vi "RSZVB Set TDIF Amplitude Imbalance Stop Power.vi"(8 "error in (no error)":errorcluster {"code" format="%.0x"}, 9 "Stop Power (+10.0 dBm)":dbl=10.0 format="%^.3e", 10 "Channel (1)":i32=1, 11 "VISA session":refnum<visa-resource-name>) -> (0 "error out":errorcluster {"code" format="%.0x"}, 3 "dup VISA session":refnum<visa-resource-name>)   [LabVIEW 2011]
doc: "This VI defines the stop power for an amplitude imbalance sweep, which is equal to the right edge of a Cartesian diagram. A balanced port configuration must be defined and an amplitude imbalance sweep must be active to use this VI.\n\nNote(s):\n\n(1) This VI is available only with option R&S ZVA-K6.\n\nRemote-control command(s):\nSOURce<Ch>:TDIF:IMBalance:AMPLitude:STOP <stop_power>"
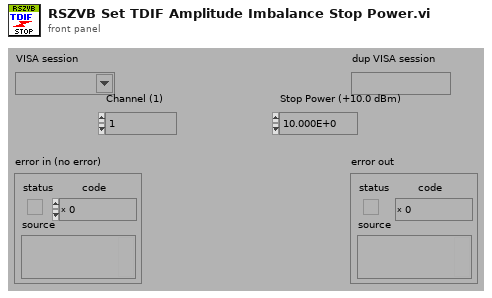
[diagram p1: front panel]
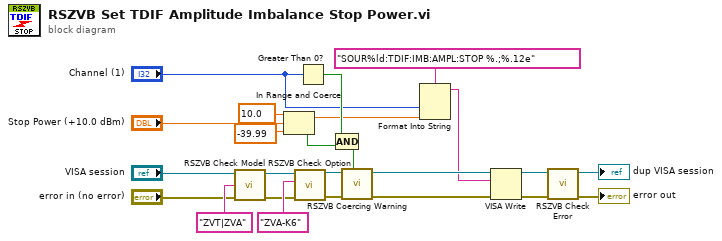
[diagram p0: block diagram]
diagram:
  n1 = call "RSZVB Check Model.vi"("error in (no error)"="error in (no error)", "Model"="ZVT|ZVA" ("Options"), "VISA session"="VISA session") -> ("error out"=w21:errorcluster, "dup VISA session"=w22:refnum<visa-resource-name>)  [unwired: 7 in]
  n2 = In Range and Coerce(upper limit=10.0, x="Stop Power (+10.0 dBm)", lower limit=-39.99) -> (coerced(x)=w9:dbl, In Range?=w16:bool)
  n3 = call "RSZVB Check Option.vi"("error in (no error)"=w21, "Options"="ZVA-K6", "VISA session"=w22) -> ("error out"=w8:errorcluster, "dup VISA session"=w7:refnum<visa-resource-name>)  [unwired: 7 in]
  n4 = Greater Than 0?(x="Channel (1)") -> (x > 0?=w15:bool)
  n5 = Compound Arithmetic op=AND(w15, w16) -> (w14:bool)
  n6 = call "RSZVB Coercing Warning.vi"("In Range?"=w14, "error in (no error)"=w8, "VISA session"=w7) -> ("error out"=w19:errorcluster, "dup VISA session"=w20:refnum<visa-resource-name>)  [unwired: 7 in]
  n7 = Format Into String(format string="SOUR%ld:TDIF:IMB:AMPL:STOP %.;%.12e", "Channel (1)", w9) -> (resulting string=w10:string)  [unwired: 2 in, 1 out]
  n8 = VISA Write(VISA resource name=w20, write buffer=w10, error in (no error)=w19) -> (VISA resource name out=w17:refnum<visa-resource-name>, error out=w18:errorcluster)  [unwired: 1 out]
  n9 = call "RSZVB Check Error.vi"("error in (no error)"=w18, "VISA session"=w17) -> ("error out"=→"error out":errorcluster, "dup VISA session"=→"dup VISA session":refnum<visa-resource-name>)  [unwired: 8 in]
